vi "Pump Status.vi"(8 "error in (no error)":errorcluster, 11 "FLOM Settings In":T1) -> (0 "error out":errorcluster, 1 "Connection Error":bool, 2 "Pump On?":enum16{"Off", "On", "Not Initialized"}(ring), 3 "FLOM Settings Out":T1={"VISA resource name"="", "Simulated?"=TRUE, "Pump Number"=0.0}, 4 "Pressure":dbl, 5 "Flow Rate":dbl)   [LabVIEW 2018, in "FLOM Pump.lvlib"]
uses:
  FLOM Pump.lvlib
  Settings Cluster.ctl
  <vilib>/Instr/_visa.llb/VISA Flush IO Buffer Mask.ctl
  <vilib>/Instr/_visa.llb/VISA Configure Serial Port (Instr).vi
  <vilib>/regexp/Match Regular Expression.xnode
panel:
  out "concatenated string":string
  out "read buffer":string
  out "result string":string
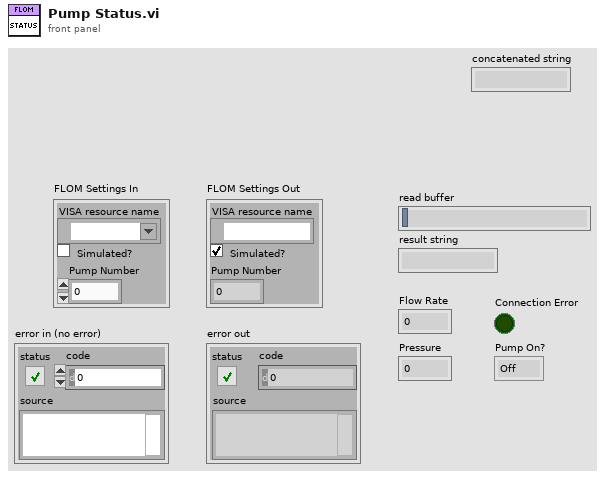
[diagram p1: front panel]
types:
  T1 = typedef "FLOM Pump.lvlib/Settings Cluster.ctl" = cluster{"VISA resource name":refnum<visa-resource-name>, "Simulated?":bool, "Pump Number":dbl}
  T2 = typedef "VISA Flush IO Buffer Mask.ctl" = u16
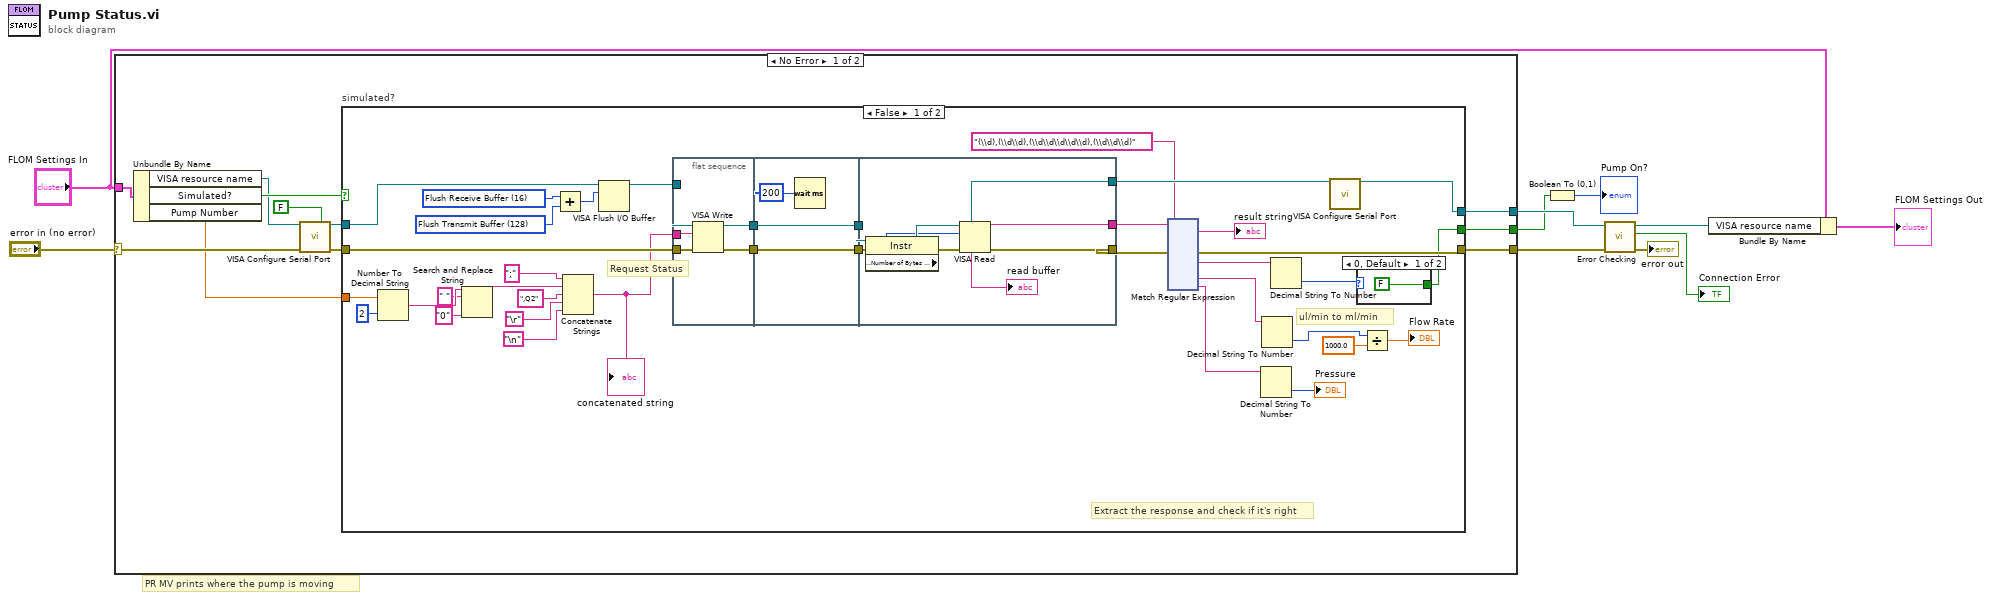
[diagram p0: block diagram]
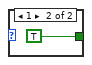
[diagram p2: hidden frame]
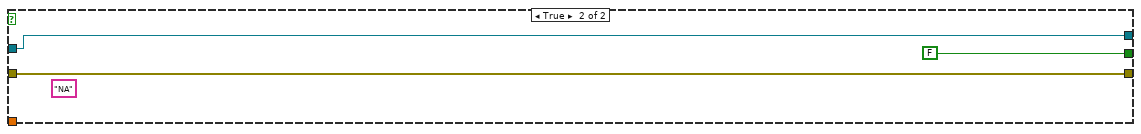
[diagram p3: hidden frame]
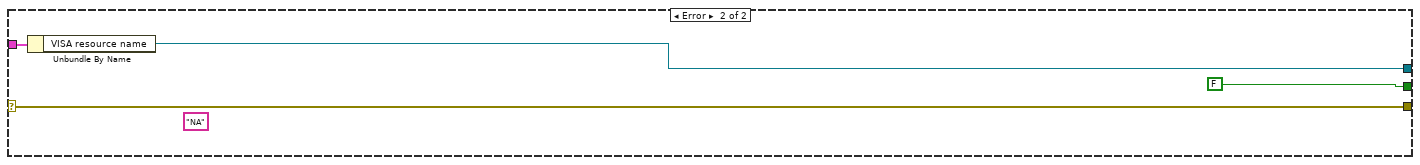
[diagram p4: hidden frame]
diagram:
  # "PR MV prints where the pump is moving"
  n1 = case shown="No Error" "error in (no error)" {
    selector: "error in (no error)" -> [w14 w202]
    tunnel: [w21 w202] -> w8
    tunnel: "FLOM Settings In" -> [w20 w201]
    tunnel: [w19 w200] -> w6
    tunnel: [w12 FALSE] -> w3
    frame No Error {
      n2 = Unbundle By Name(w20) -> ("VISA resource name"=w17:refnum<visa-resource-name>, "Simulated?"=w18:bool, "Pump Number"=w11:dbl)
      n3 = call-poly "VISA Configure Serial Port"("VISA resource name"=w17, "Enable Termination\nChar (T)"=FALSE ("Enable Termination\nChar (T)"), "error in (no error)"=w14) -> ("VISA resource name out"=w16:refnum<visa-resource-name>, "error out"=w13:errorcluster)  [unwired: 11 in]
      n4 = case "simulated?" shown="False" w18 {
        tunnel: [w38 w198] -> w21
        tunnel: [w47 w196] -> w19
        tunnel: w13 -> [w58 w198]
        tunnel: w16 -> [w53 w196]
        tunnel: [w35 FALSE] -> w12
        tunnel: w11 -> [w26 _]
        frame False {
          w49 = T2 128 items=["Flush Receive Buffer"=16, "Write Transmit Buffer to Device"=32, "Flush Receive Buffer (No I/O)"=64, "Flush Transmit Buffer"=128] ("Mask")
          w50 = T2 16 items=["Flush Receive Buffer"=16, "Write Transmit Buffer to Device"=32, "Flush Receive Buffer (No I/O)"=64, "Flush Transmit Buffer"=128] ("Mask")
          # "ul/min to ml/min"
          # "Extract the response and check if it's right"
          # "Request Status"
          n5 = Number To Decimal String(number=w26, width (-)=i16 2) -> (decimal integer string=w29:string)
          n6 = Search and Replace String(input string=w29, search string=" ", replace string="0" ("replace string (\"\")")) -> (result string=w25:string)  [unwired: 5 in, 3 out]
          n7 = Add(x=w50, y=w49) -> (x+y=w51:T2)
          n8 = Concatenate Strings(";" ("string"), w25, ",Q2" ("string"), "\r", "\n") -> (w42:string)
          "concatenated string" <- w42
          n9 = VISA Flush I/O Buffer(VISA resource name=w53, mask (16)=w51) -> (VISA resource name out=w52:refnum<visa-resource-name>)  [unwired: 1 in, 1 out]
          n10 = flat-sequence {
            tunnel: [w183] -> w57
            tunnel: [w184] -> w56
            tunnel: w58 -> [w181]
            tunnel: w52 -> [w182]
            tunnel: w42 -> [w180]
            tunnel: w57 -> [w185]
            tunnel: w56 -> [w187]
            tunnel: [w187] -> w55
            tunnel: [w185] -> w54
            tunnel: w55 -> [w195]
            tunnel: w54 -> [w194]
            tunnel: [w190] -> w41
            tunnel: [w189] -> w48
            tunnel: [w188] -> w40
            frame #0 {
              n11 = VISA Write(VISA resource name=w182, write buffer=w180, error in (no error)=w181) -> (VISA resource name out=w183:refnum<visa-resource-name>, error out=w184:errorcluster)  [unwired: 1 out]
            }
            frame #1 {
              n12 = Wait (ms)(milliseconds to wait=u32 200) -> ()  [unwired: 1 out]
            }
            frame #2 {
              n13 = property class="Instr"(reference=w194, error in=w195) -> (reference out=w193:refnum<visa-resource-name>, error out=w192:errorcluster, "Serial Settings:Number of Bytes at Serial Port"=w191:u32)
              n14 = VISA Read(VISA resource name=w193, byte count=w191, error in (no error)=w192) -> (VISA resource name out=w189:refnum<visa-resource-name>, read buffer=w190:string, error out=w188:errorcluster)  [unwired: 1 out]
              "read buffer" <- w190
            }
          }
          n15 = xnode "Match Regular Expression"("input string"=w41, "regular expression"="(\\d),(\\d\\d),(\\d\\d\\d\\d\\d),(\\d\\d\\d)", "error in"=w40) -> ("whole match"=→"result string":string, "error out"=w38:errorcluster, "submatch 1"=w37:string, "submatch 3"=w33:string, "submatch 4"=w32:string)  [unwired: 3 in, 4 out]
          n16 = Decimal String To Number(string=w32) -> (number=→"Pressure":i32)  [unwired: 2 in, 1 out]
          n17 = Decimal String To Number(string=w33) -> (number=w22:i32)  [unwired: 2 in, 1 out]
          n18 = Decimal String To Number(string=w37) -> (number=w36:i32)  [unwired: 2 in, 1 out]
          n19 = call-poly "VISA Configure Serial Port"("VISA resource name"=w48) -> ("VISA resource name out"=w47:refnum<visa-resource-name>)  [unwired: 13 in, 1 out]
          n20 = case shown="0, Default" w36 {
            tunnel: [FALSE TRUE] -> w35
            frame 0, Default {
            }
            frame 1 {
            }
          }
          n21 = Divide(x=w22, y=1000.0) -> (x/y=→"Flow Rate":dbl)
        }
        frame True {
          (unwired) "NA" ("read buffer")
        }
      }
    }
    frame Error {
      (unwired) "NA" ("read buffer")
      n22 = Unbundle By Name(w201) -> ("VISA resource name"=w200:refnum<visa-resource-name>)
    }
  }
  n23 = Boolean To (0,1)(Boolean=w3) -> (0, 1=→"Pump On?":i16)
  n24 = call "Error Checking.vi"("error in (no error)"=w8, "VISA resource name"=w6) -> ("error out"=→"error out":errorcluster, "Connection Error"=→"Connection Error":bool, "VISA resource name"=w5:refnum<visa-resource-name>)  [unwired: 7 in]
  n25 = Bundle By Name(cluster="FLOM Settings In", "VISA resource name"=w5) -> (→"FLOM Settings Out":T1)
